vi "Specify ARN Tag.vi"(11 "Endpoint in":refnum<class "Endpoint.lvclass">) -> (2 "ARN Tag":string, 3 "Endpoint out":refnum<class "Endpoint.lvclass">)   [LabVIEW 2015, in "NI_AWS_SNS.lvlib" / "Endpoint.lvclass"]
uses:
  Endpoint.lvclass
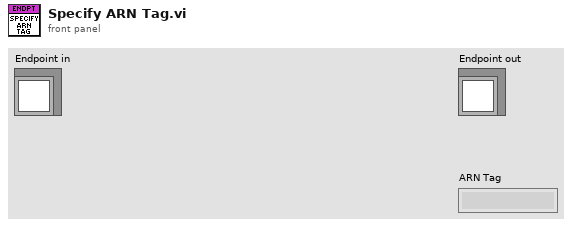
[diagram p1: front panel]
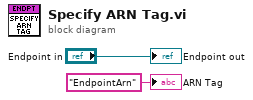
[diagram p0: block diagram]
diagram:
  "Endpoint out" <- "Endpoint in"
  "ARN Tag" <- "EndpointArn" ("ARN Tag")
